vi "要求值到报表.vi"(8 "错误输入（无错误）":errorcluster caption="error out", 9 "refnum":T1, 10 "error out":errorcluster, 11 "引用句柄输入":T1 caption="refnum") -> (0 "错误输出":errorcluster caption="error out", 1 "error out 3":errorcluster caption="error out", 2 "refnum out":T1, 3 "引用句柄输出":T1 caption="refnum out")   [LabVIEW 2013]
doc: "把要求值表格中的一些固定参数读到油动机报表"
uses:
  <vilib>/Utility/config.llb/Config Data RefNum.ctl
  <vilib>/Utility/config.llb/Read Key (String).vi
  <vilib>/Utility/config.llb/Write Key (String).vi
  <vilib>/Utility/config.llb/NI_LVConfig.lvlib
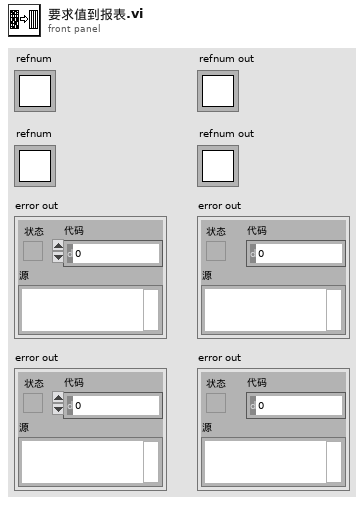
[diagram p1: front panel]
types:
  T1 = typedef "NI_LVConfig.lvlib/Config Data RefNum.ctl" = refnum<k1>
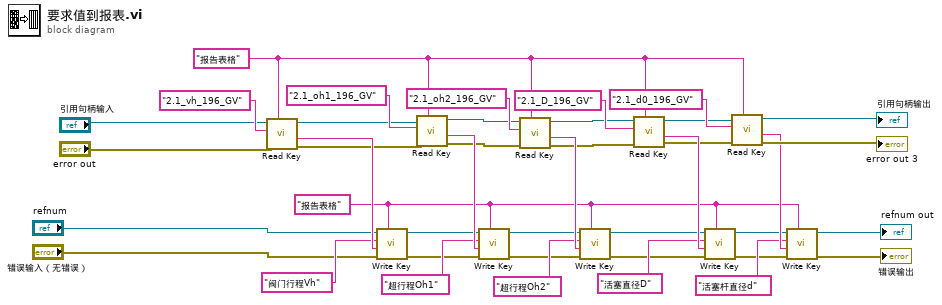
[diagram p0: block diagram]
diagram:
  w14 = "报告表格" ("section")
  w28 = "报告表格" ("section")
  n1 = call-poly <vilib>:"Read Key.vi"("section"=w28, "error in (no error)"="error out", "key"="2.1_vh_196_GV", "refnum"="引用句柄输入") -> ("error out"=w19:errorcluster, "value"=w27:string, "refnum out"=w20:T1)  [unwired: 4 in, 1 out]
  n2 = call-poly <vilib>:"Write Key.vi"("section"=w14, "error in (no error)"="错误输入（无错误）", "value"=w27, "key"="阀门行程Vh", "refnum"="refnum") -> ("error out"=w6:errorcluster, "refnum out"=w7:T1)  [unwired: 4 in, 1 out]
  n3 = call-poly <vilib>:"Read Key.vi"("section"=w28, "error in (no error)"=w19, "key"="2.1_oh1_196_GV" ("default value"), "refnum"=w20) -> ("error out"=w21:errorcluster, "value"=w30:string, "refnum out"=w22:T1)  [unwired: 4 in, 1 out]
  n4 = call-poly <vilib>:"Write Key.vi"("section"=w14, "error in (no error)"=w6, "value"=w30, "key"="超行程Oh1", "refnum"=w7) -> ("error out"=w8:errorcluster, "refnum out"=w9:T1)  [unwired: 4 in, 1 out]
  n5 = call-poly <vilib>:"Read Key.vi"("section"=w28, "error in (no error)"=w21, "key"="2.1_oh2_196_GV", "refnum"=w22) -> ("error out"=w23:errorcluster, "value"=w32:string, "refnum out"=w24:T1)  [unwired: 4 in, 1 out]
  n6 = call-poly <vilib>:"Write Key.vi"("section"=w14, "error in (no error)"=w8, "value"=w32, "key"="超行程Oh2", "refnum"=w9) -> ("error out"=w10:errorcluster, "refnum out"=w11:T1)  [unwired: 4 in, 1 out]
  n7 = call-poly <vilib>:"Read Key.vi"("section"=w28, "error in (no error)"=w23, "key"="2.1_D_196_GV", "refnum"=w24) -> ("error out"=w26:errorcluster, "value"=w34:string, "refnum out"=w25:T1)  [unwired: 4 in, 1 out]
  n8 = call-poly <vilib>:"Write Key.vi"("section"=w14, "error in (no error)"=w10, "value"=w34, "key"="活塞直径D", "refnum"=w11) -> ("error out"=w12:errorcluster, "refnum out"=w13:T1)  [unwired: 4 in, 1 out]
  n9 = call-poly <vilib>:"Read Key.vi"("section"=w28, "error in (no error)"=w26, "key"="2.1_d0_196_GV", "refnum"=w25) -> ("error out"=→"error out 3":errorcluster, "value"=w36:string, "refnum out"=→"引用句柄输出":T1)  [unwired: 4 in, 1 out]
  n10 = call-poly <vilib>:"Write Key.vi"("section"=w14, "error in (no error)"=w12, "value"=w36, "key"="活塞杆直径d", "refnum"=w13) -> ("error out"=→"错误输出":errorcluster, "refnum out"=→"refnum out":T1)  [unwired: 4 in, 1 out]
